vi "LinearFilter_HighPassBW2.vi"(9 "SamplePeriod":dbl format="%13.5p", 11 "TimeConstant":dbl format="%13.5p") -> (3 "LINEAR_FILTER":T1 {"Outputs" format="%13.5g"; "Inputs" format="%13.5g"; "OutputGains" format="%13.5g"; "InputGains" format="%13.5g"})   [LabVIEW 2023]
doc: "Creates a 2nd order Butterworth high pass filter.\n\nA 2nd order filter provides more filtering, however it also has a larger phase shift (time delay).\n\nMore information on this type of filter can be found at:\n\n https://en.wikipedia.org/wiki/Butterworth_filter\n\nInputs: \n - timeConstant - The discrete-time time constant in seconds.\n - samplePeriod - The period in seconds between samples taken by the user.\n\nOutputs:\n - Linearfilter - Created datat structure"
uses:
  <vilib>/Rock Robotics/WPI/ThirdParty/JAS_Junk/TrajLib/TypeDef/LINEAR_FILTER.ctl
  <vilib>/Rock Robotics/SystemInterfaces/NetworkCommunication/NetComm_UsageReport_report.vi
  <vilib>/Rock Robotics/WPI/ThirdParty/JAS_Junk/TrajLib/Globals/Util_LibraryGlobals.vi
  <vilib>/Rock Robotics/WPI/ThirdParty/JAS_Junk/TrajLib/Trajectory_Library.lvlib
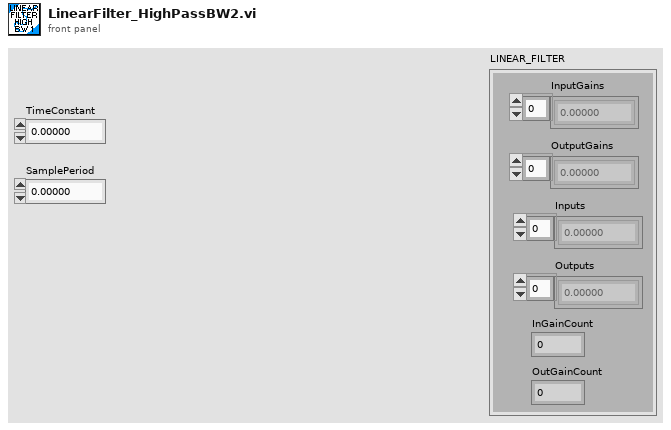
[diagram p1: front panel]
types:
  T1 = typedef "Trajectory_Library.lvlib/LINEAR_FILTER.ctl" = cluster{"InputGains":dbl[], "OutputGains":dbl[], "Inputs":dbl[], "Outputs":dbl[], "InGainCount":i32, "OutGainCount":i32}
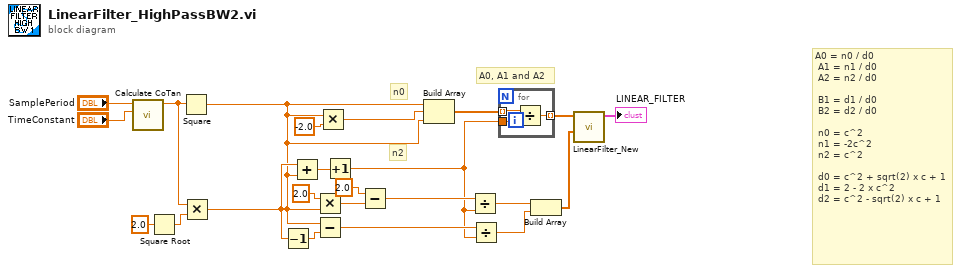
[diagram p0: block diagram]
diagram:
  # "n2"
  # "n0"
  # "A0, A1 and A2"
  # "A0 = n0 / d0\n\tA1 = n1 / d0\n\tA2 = n2 / d0\n\n\tB1 = d1 / d0\n\tB2 = d2 / d0\n\n\tn0 = c^2\n\tn1 = -2c^2\n n2 = c^2\n\n\td0 = c^2 + sqrt(2) x c + 1\n\td1 = 2 - 2 x c^2\n\td2 = c^2 - sqrt(2) x c + 1"
  n1 = call "Calculate CoTan.vi"("TimeConstant (sec)"="TimeConstant", "SamplePeriod (sec)"="SamplePeriod") -> ("C"=w21:dbl)  [unwired: 8 in, 1 out]
  n2 = Square Root(x=2.0) -> (sqrt(x)=w22:dbl)
  n3 = Square(x=w21) -> (x^2=w8:dbl)
  n4 = Multiply(x=w21, y=w22) -> (x*y=w13:dbl)
  n5 = Decrement(x=w13) -> (x-1=w16:dbl)
  n6 = Add(x=w13, y=w8) -> (x+y=w20:dbl)
  n7 = Multiply(x=2.0, y=w8) -> (x*y=w18:dbl)
  n8 = Subtract(x=w8, y=w16) -> (x-y=w11:dbl)
  n9 = Multiply(x=w8, y=-2.0) -> (x*y=w9:dbl)
  n10 = Increment(x=w20) -> (x+1=w6:dbl)
  n11 = Subtract(x=2.0 ("y"), y=w18) -> (x-y=w12:dbl)
  n12 = Build Array(w8, w9, w8) -> (w7:dbl[])
  n13 = Divide(x=w12, y=w6) -> (x/y=w5:dbl)
  n14 = Divide(x=w11, y=w6) -> (x/y=w4:dbl)
  n15 = for {
    tunnel: w7 -> [w26] mode=indexing
    tunnel: w6 -> [w25]
    tunnel: [w24] -> w2 mode=indexing
    n16 = Divide(x=w26, y=w25) -> (x/y=w24:dbl)
  }
  n17 = Build Array(w5, w4) -> (w1:dbl[])
  n18 = call <vilib>:"LinearFilter_New.vi"("OutputGains"=w1, "InputGains"=w2) -> ("LINEAR_FILTER"=→"LINEAR_FILTER":T1)  [unwired: 9 in]
